vi "Initialise bleaching compensation.vi"(8 "error in (no error)":errorcluster, 11 "RSA in":refnum<class "RSA.lvclass">) -> (0 "error out":errorcluster, 3 "RSA out":refnum<class "RSA.lvclass">)   [LabVIEW 2012, in "RSA.lvclass"]
uses:
  RSA.lvclass
  <vilib>/Distrio/Murmex/GenericMessage/GenericMessage.lvclass
  <vilib>/Distrio/Murmex/Message/Add or replace parameter.vi
  <vilib>/Distrio/Murmex/Murmex/Murmex.lvclass
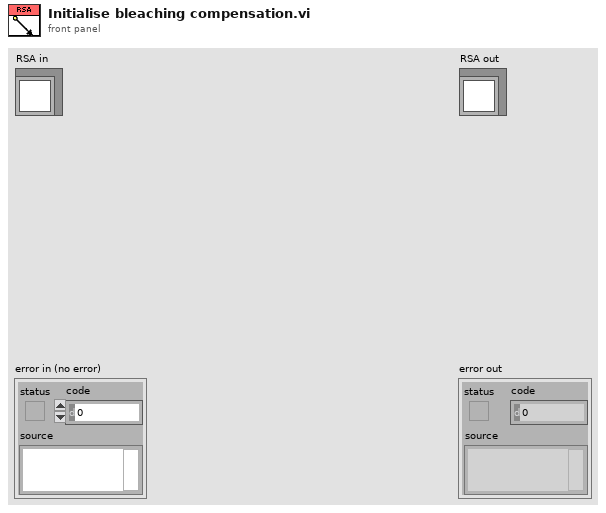
[diagram p1: front panel]
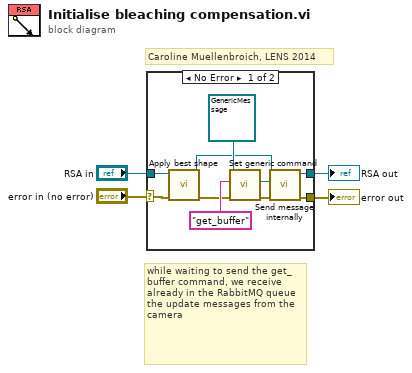
[diagram p0: block diagram]
diagram:
  # "while waiting to send the get_buffer command, we receive already in the RabbitMQ queue the update messages from the camera"
  # "Caroline Muellenbroich, LENS 2014"
  n1 = case shown="No Error" "error in (no error)" {
    selector: "error in (no error)" -> [w8 w16]
    tunnel: [w11 w16] -> w3
    tunnel: [w10 w15] -> w1
    tunnel: "RSA in" -> [w6 w15]
    frame No Error {
      n2 = call "Apply best shape.vi"("error in (no error)"=w8, "RSA in"=w6) -> ("error out"=w7:errorcluster, "RSA out"=w5:refnum<class "RSA.lvclass">)  [unwired: 8 in]
      n3 = call <vilib>:"Set generic command.vi"("error in (no error)"=w7, "generic command"="get_buffer", "GenericMessage in"=refnum<class "GenericMessage.lvclass"> refnum ("Murmex.lvlib:GenericMessage")) -> ("error out"=w13:errorcluster, "GenericMessage out"=w14:refnum<class "GenericMessage.lvclass">)  [unwired: 7 in]
      n4 = call <vilib>:"Send message internally.vi"("error in (no error)"=w13, "Message"=w14, "Murmex in"=w5) -> ("error out"=w11:errorcluster, "Murmex out"=w10:refnum<class "RSA.lvclass">)  [unwired: 7 in]
    }
    frame Error {
    }
  }
  "error out" <- w3
  "RSA out" <- w1
